vi "ArrayRemove_I.vi"(7 "N":i32 min=0, 10 "To Remove":i32, 11 "1D Array In":i32[](array[numeric])) -> (0 "1D Array Out":i32[](array[numeric]), 3 "Removed All":bool)   [LabVIEW 2009]
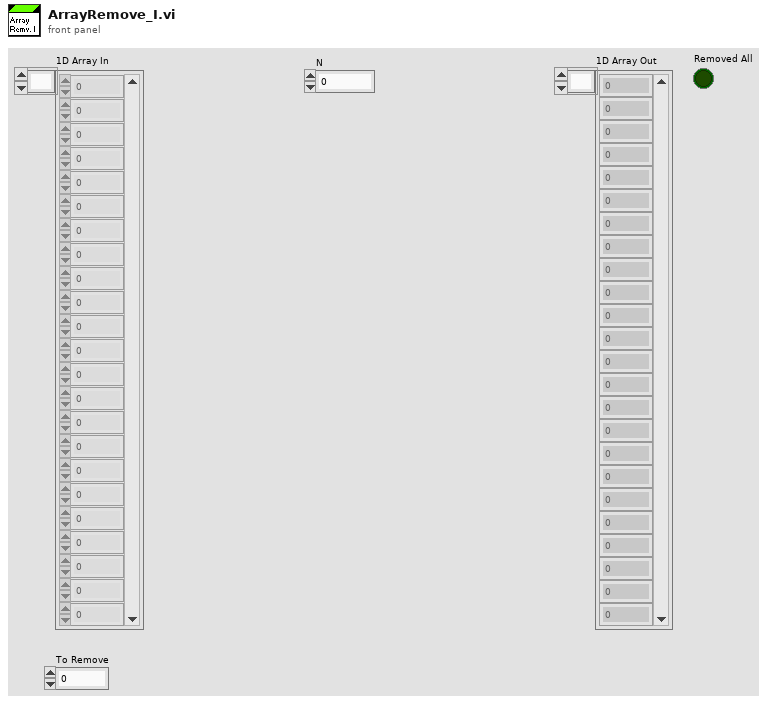
[diagram p1: front panel]
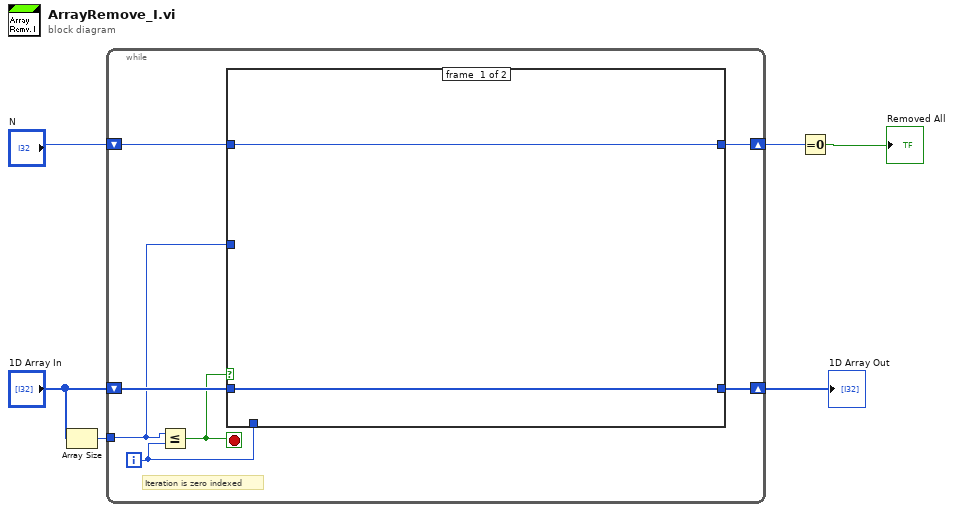
[diagram p0: block diagram]
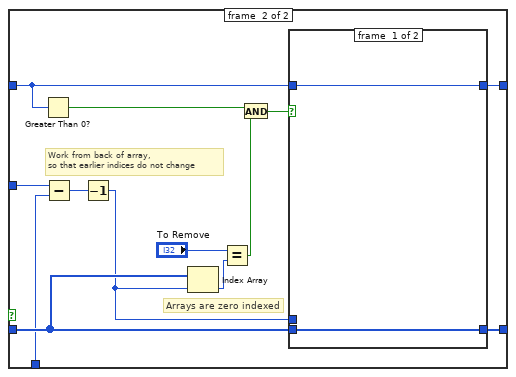
[diagram p2: hidden frame]
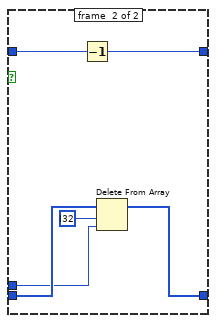
[diagram p3: hidden frame]
diagram:
  n1 = Array Size(array="1D Array In") -> (size(s)=w6:i32)
  n2 = while {
    tunnel: w6 -> [w7]
    shift-right: [w11] -> w4
    shift-left: "1D Array In" -> [w13]
    shift-right: [w8] -> w2
    shift-left: "N" -> [w9]
    i -> [w12]
    stop <- w10 stop-if-true
    # "Iteration is zero indexed"
    n3 = Less Or Equal?(x=w7, y=w12) -> (x <= y?=w10:bool)
    n4 = case shown="False" w10 {
      tunnel: w13 -> [w15 w26]
      tunnel: w12 -> [_ w18]
      tunnel: [w15 w25] -> w11
      tunnel: w9 -> [w14 w21]
      tunnel: [w14 w20] -> w8
      tunnel: w7 -> [_ w19]
      frame #0 {
      }
      frame #1 {
        # "Arrays are zero indexed"
        # "Work from back of array,\nso that earlier indices do not change"
        n5 = Greater Than 0?(x=w21) -> (x > 0?=w22:bool)
        n6 = Subtract(x=w19, y=w18) -> (x-y=w17:i32)
        n7 = Decrement(x=w17) -> (x-1=w16:i32)
        n8 = Index Array(array=w26, index=w16) -> (element=w28:i32)
        n9 = Equal?(x="To Remove", y=w28) -> (x = y?=w24:bool)
        n10 = And(x=w22, y=w24) -> (x .and. y?=w23:bool)
        n11 = case shown="True" w23 {
          tunnel: w26 -> [w30 w36]
          tunnel: w16 -> [_ w34]
          tunnel: [w30 w33] -> w25
          tunnel: w21 -> [w29 w32]
          tunnel: [w29 w31] -> w20
          frame #0 {
          }
          frame #1 {
            n12 = Decrement(x=w32) -> (x-1=w31:i32)
            n13 = Delete From Array(array=w36, length=i32 ?, index=w34) -> (array with subset deleted=w33:i32[])  [unwired: 1 out]
          }
        }
      }
    }
  }
  "1D Array Out" <- w4
  n14 = Equal To 0?(x=w2) -> (x = 0?=→"Removed All":bool)
